vi "Shutdown.vi"(8 "error in":errorcluster, 11 "User Interface Control Reference":refnum<queue>) -> (0 "error out":errorcluster)   [LabVIEW 2011]
uses:
  Controls/User Interface Control.ctl
  Controls/User Interface Action.ctl
  Functional Globals/User Interface Global Action.ctl
  Modules/Menu/Menu Action.ctl
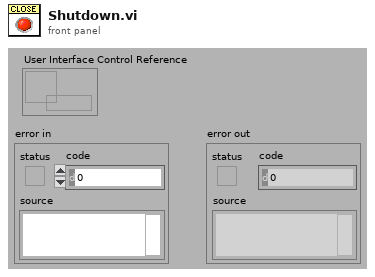
[diagram p1: front panel]
types:
  T1 = typedef "User Interface Global Action.ctl" = enum16{"Initialize", "Update UI", "Stop"}
  T2 = typedef "User Interface Action.ctl" = enum16{"Initialize", "Update Real Channel", "Update Imag Channel", "Update Re/Im channel @ Hardware Ctrl", "Pulse Sequence", "Visibility Front Panel Controls", "Report Custom Errors", "Set Pulse Sequence Type", "Update Pulse Timings", "Update Transfer Time", "Update Status Bar", "Set Sequence Progress", "Set 90 Degree Pulse Sequence Params", "Set CMPG Pulse Sequence Parms", "Set T1 Pulse Sequence Params", "Stop"}
  T3 = typedef "Menu Action.ctl" = enum16{"Initialize", "Insert Item", "Remove Item", "Set Checked Item", "Get Checked Item", "Get Item Index", "Item Present?", "Stop"}
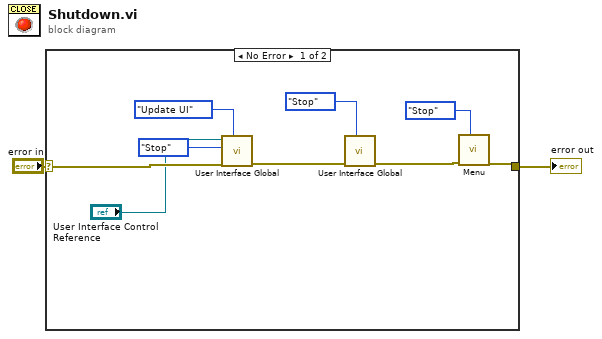
[diagram p0: block diagram]
diagram:
  n1 = case shown="No Error" "error in" {
    selector: "error in" -> [w9 w12]
    tunnel: [w11 w12] -> w1
    frame No Error {
      n2 = call "User Interface Global.vi"("command (Update UI)"=User_Interface_Global_Action."Update UI", "error in"=w9, "action"=User_Interface_Action."Stop", "user interface queue reference"="User Interface Control Reference") -> ("error out"=w5:errorcluster)  [unwired: 7 in]
      n3 = call "User Interface Global.vi"("command (Update UI)"=User_Interface_Global_Action."Stop", "error in"=w5) -> ("error out"=w4:errorcluster)  [unwired: 9 in]
      n4 = call "Menu.vi"("action"=Menu_Action."Stop" ("Menu"), "error in"=w4) -> ("error out"=w11:errorcluster)  [unwired: 6 in, 3 out]
    }
    frame Error {
    }
  }
  "error out" <- w1
